vi "Sandbox - Add VI to Project.vi"(8 "error in":errorcluster) -> (0 "error out":errorcluster)   [LabVIEW 2020]
doc: "Sandbox"
panel:
  out "Type String":string
  out "Owner Type String":string
  out "OwnedItems Type String":string[](array[string])
  out "index of element":i32
  out "Projects":string[](array[string])
  in  "Project Name":string
  in  "References of In-Memory Projects":refnum<vi>[](array[refnum])
  in  "Reference of newly created VI":refnum<vi>
  out "error out 2":errorcluster
  in  "error in 2":errorcluster
  # "Development\ncontrols/indicators useful for development and testing, but which are not outputs of the VI"
  # "Input\nInputs to the VI"
  # "Output\nOutputs of the VI"
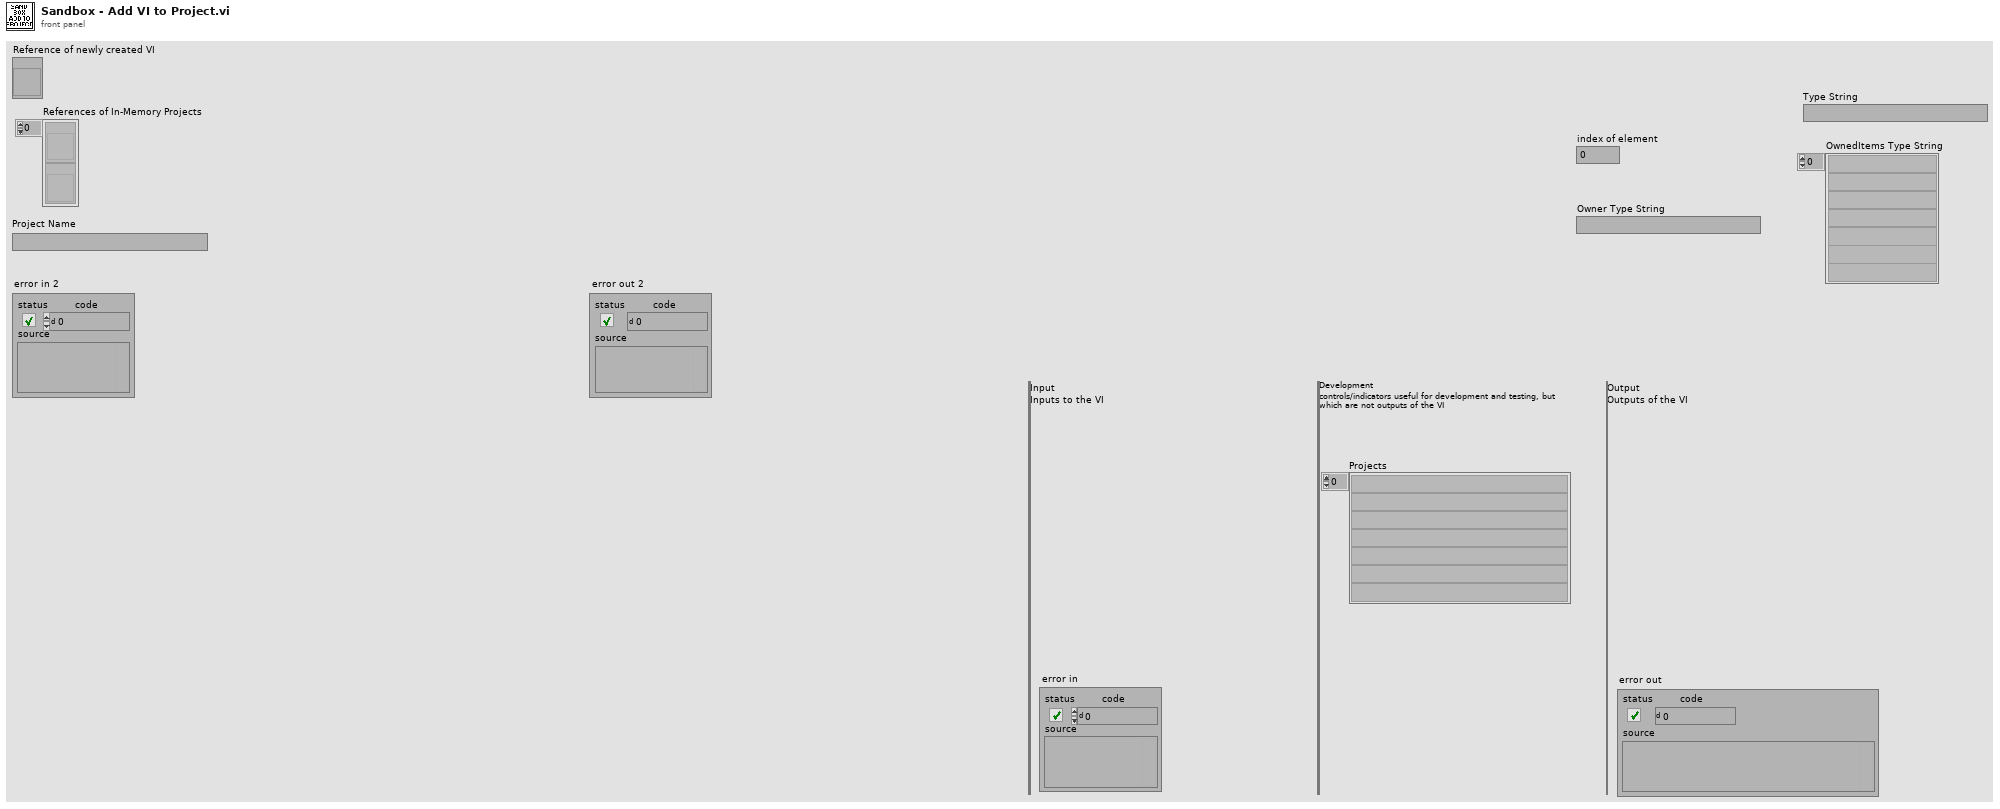
[diagram p1: front panel]
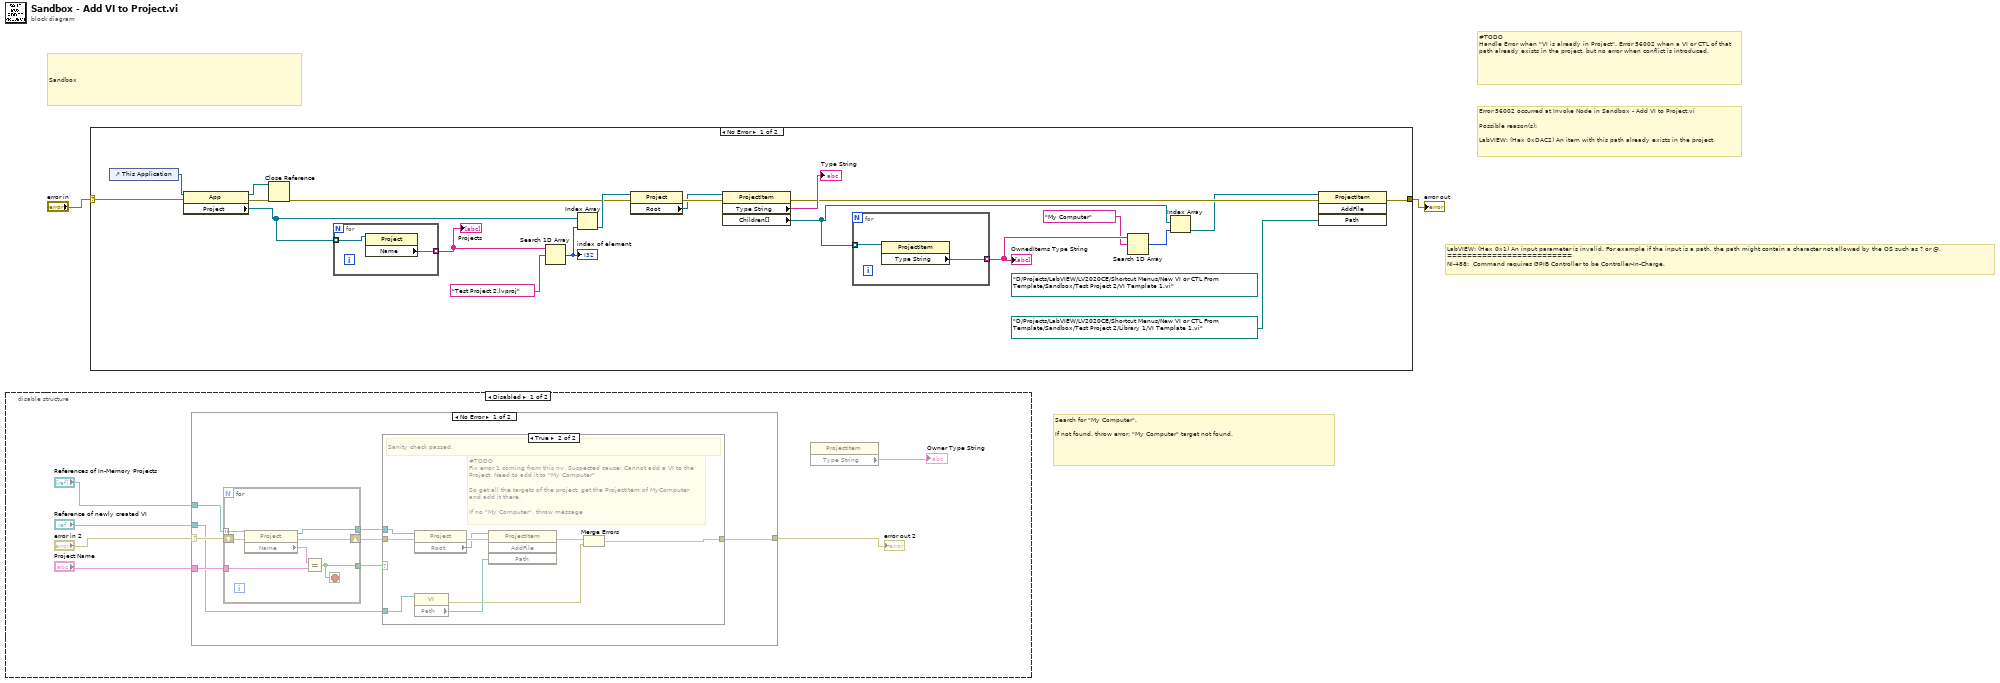
[diagram p0: block diagram]
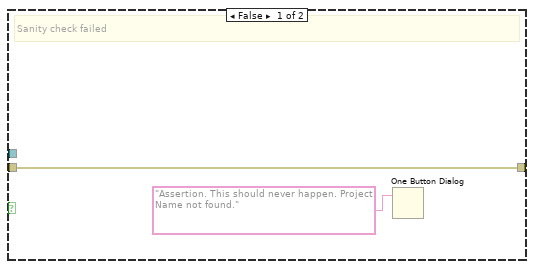
[diagram p3: hidden frame]
diagram:
  # "Error 56002 occurred at Invoke Node in Sandbox - Add VI to Project.vi\n\nPossible reason(s):\n\nLabVIEW: (Hex 0xDAC2) An item with this path already exists in the project."
  # "LabVIEW: (Hex 0x1) An input parameter is invalid. For example if the input is a path, the path might contain a character not allowed by the OS such as ? or @.\n=========================\nNI-488:  Command requires GPIB Controller to be Controller-In-Charge."
  # "Search for \"My Computer\".\n\nIf not found, throw error: \"My Computer\" target not found."
  # "#TODO\nHandle Error when \"VI is already in Project\". Error 56002 when a VI or CTL of that path already exists in the project, but no error when conflict is introduced."
  # "Sandbox"
  n1 = disable-structure shown="Disabled" {
    frame Disabled {
      n2 = case shown="No Error" "error in 2" {
        selector: "error in 2" -> [w16 w36]
        tunnel: [w17 w36] -> w8
        tunnel: "References of In-Memory Projects" -> [w15 _]
        tunnel: "Reference of newly created VI" -> [w10 _]
        tunnel: "Project Name" -> [w14 _]
        frame No Error {
          n3 = for {
            shift-right: [w23] -> w13
            shift-left: w16 -> [w24]
            tunnel: w15 -> [w22] mode=indexing
            tunnel: w14 -> [w20]
            tunnel: [w19] -> w12
            tunnel: [w18] -> w11
            stop <- w19 stop-if-true
            n4 = property class="Project"(reference=w22, error in=w24) -> (reference out=w18:refnum<vi>, error out=w23:errorcluster, "Name"=w21:string)
            n5 = Equal?(x=w21, y=w20) -> (x = y?=w19:bool)
          }
          n6 = case shown="True" w12 {
            tunnel: [w26 w28] -> w17
            tunnel: w13 -> [w26 w35]
            tunnel: w11 -> [_ w33]
            tunnel: w10 -> [_ w30]
            frame False {
              # "Sanity check failed"
              n7 = One Button Dialog(message="Assertion. This should never happen. Project Name not found.") -> ()  [unwired: 1 in, 1 out]
            }
            frame True {
              # "#TODO\nFix error 1 coming from this nv. Suspected cause: Cannot add a VI to the Project. Need to add it to \"My Computer\"\n\nSo get all the targets of the project, get the ProjectItem of MyComputer and add it there.\n\nIf no \"My Computer\", throw message"
              # "Sanity check passed."
              n8 = property class="Project"(reference=w33, error in=w35) -> (error out=w34:errorcluster, "Root"=w31:refnum<vi>)  [unwired: 1 out]
              n9 = property class="VI"(reference=w30) -> (error out=w27:errorcluster, "Path"=w29:path)  [unwired: 1 in, 1 out]
              n10 = invoke class="ProjectItem" method="AddFile"(reference=w31, error in=w34, "Path"=w29) -> (error out=w32:errorcluster)  [unwired: 1 in, 3 out]
              n11 = Merge Errors(w32, w27) -> (w28:errorcluster)
            }
          }
        }
        frame Error {
        }
      }
      "error out 2" <- w8
      n12 = property class="ProjectItem"() -> (error out=w4:errorcluster, "Type String"=→"Owner Type String":string)  [unwired: 2 in, 1 out]
    }
    frame Enabled {
    }
  }
  n13 = case shown="No Error" "error in" {
    selector: "error in" -> [w54 w62]
    tunnel: [w39 w62] -> w1
    frame No Error {
      (unwired) path "D:/Projects/LabVIEW/LV2020CE/Shortcut Menus/New VI or CTL From Template/Sandbox/Test Project 2/VI Template 1.vi"
      n14 = control-ref of="This Application"() -> (w56:refnum<vi>)
      n15 = property class="App"(reference=w56, error in=w54) -> (reference out=w57:refnum<vi>, error out=w55:errorcluster, "Project"=w51:refnum<vi>[])
      n16 = Close Reference(reference=w57, error in (no error)=w55) -> (error out=w48:errorcluster)
      n17 = for {
        tunnel: w51 -> [w61] mode=indexing
        tunnel: [w60] -> w53 mode=indexing
        n18 = property class="Project"(reference=w61) -> ("Name"=w60:string)  [unwired: 1 in, 2 out]
      }
      "Projects" <- w53
      n19 = Search 1D Array(1D array=w53, element="Test Project 2.lvproj") -> (index of element=w50:i32)  [unwired: 1 in]
      "index of element" <- w50
      n20 = Index Array(array=w51, index=w50) -> (element=w49:refnum<vi>)
      n21 = property class="Project"(reference=w49, error in=w48) -> (error out=w47:errorcluster, "Root"=w46:refnum<vi>)  [unwired: 1 out]
      n22 = property class="ProjectItem"(reference=w46, error in=w47) -> (error out=w40:errorcluster, "Type String"=→"Type String":string, "Children[]"=w42:refnum<vi>[])  [unwired: 1 out]
      n23 = for {
        tunnel: w42 -> [w59] mode=indexing
        tunnel: [w58] -> w44 mode=indexing
        n24 = property class="ProjectItem"(reference=w59) -> ("Type String"=w58:string)  [unwired: 1 in, 2 out]
      }
      "OwnedItems Type String" <- w44
      n25 = Search 1D Array(1D array=w44, element="My Computer") -> (index of element=w41:i32)  [unwired: 1 in]
      n26 = Index Array(array=w42, index=w41) -> (element=w38:refnum<vi>)
      n27 = invoke class="ProjectItem" method="AddFile"(reference=w38, error in=w40, "Path"=path "D:/Projects/LabVIEW/LV2020CE/Shortcut Menus/New VI or CTL From Template/Sandbox/Test Project 2/Library 1/VI Template 1.vi") -> (error out=w39:errorcluster)  [unwired: 1 in, 3 out]
    }
    frame Error {
    }
  }
  "error out" <- w1
